vi "FrameBin.vi"(9 "数值":i32, 10 "data value reference输入":refnum<data-value>, 11 "队列输入":refnum<queue>) -> (2 "data value reference输出":refnum<data-value>, 3 "队列输出":refnum<queue>)   [LabVIEW 2011]
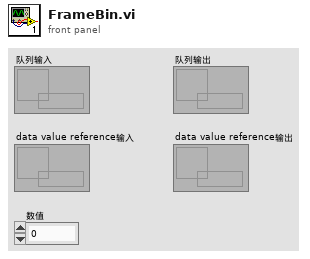
[diagram p1: front panel]
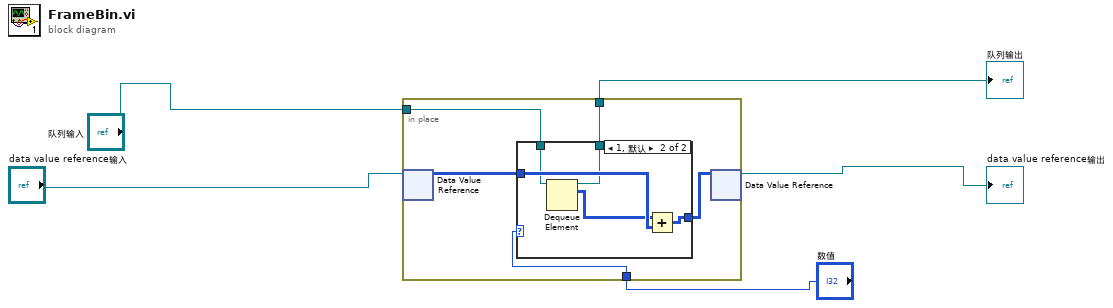
[diagram p0: block diagram]
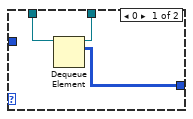
[diagram p2: hidden frame]
diagram:
  n1 = in-place {
    in-place-border: "数值" -> [w10]
    in-place-border: "队列输入" -> [w7]
    in-place-border: [w6] -> w5
    n2 = in-place-dvr #1("data value reference输入") -> (w9:u32[][])  [unwired: 1 out]
    n3 = case shown="1, 默认" w10 {
      tunnel: w9 -> [_ w18]
      tunnel: [w12 w17] -> w8
      tunnel: w7 -> [w13 w16]
      tunnel: [w11 w14] -> w6
      frame 0 {
        n4 = Dequeue Element(queue=w13) -> (queue out=w11:refnum<queue>, element=w12:i16[][])  [unwired: 2 in, 2 out]
      }
      frame 1, Default {
        n5 = Dequeue Element(queue=w16) -> (queue out=w14:refnum<queue>, element=w15:i16[][])  [unwired: 2 in, 2 out]
        n6 = Add(x=w15, y=w18) -> (x+y=w17:u32[][])
      }
    }
    n7 = in-place-dvr #1(w8) -> (→"data value reference输出":refnum<data-value>)  [unwired: 1 out]
  }
  "队列输出" <- w5
